vi "Close.vi"(8 "error in (no error)":errorcluster, 11 "LXIPXISwitching in":refnum<class "LXIPXISwitching.lvclass">) -> (0 "error out":errorcluster, 3 "LXIPXISwitching out":refnum<class "LXIPXISwitching.lvclass">)   [LabVIEW 2019, in "LXIPXISwitching.lvclass"]
uses:
  LXIPXISwitching.lvclass
  InstrumentSetup.vi
  InstrControl.lvclass
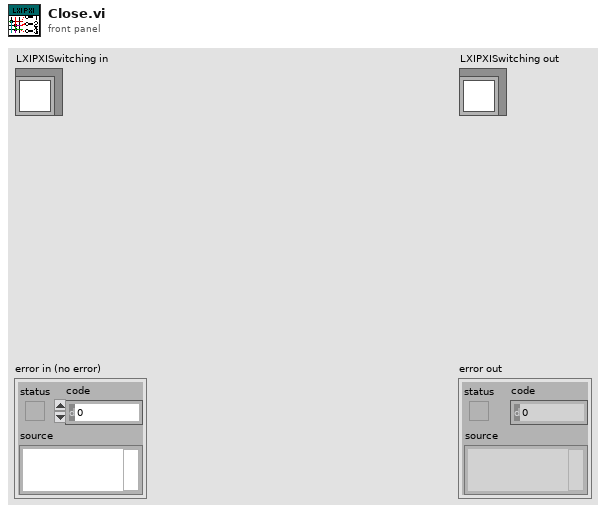
[diagram p1: front panel]
types:
  T1 = cluster{"MUX":string, "Matrix":string, "Breadboard":string, "LXIPXI Switching":refnum<class "LXIPXISwitching.lvclass">, "MUX PN":string, "Matrix  PN":string, "Breadboard PN":string, "MUX ID":string, "Matrix ID":string, "Breadboard ID":string, "LCR?":bool, "SMU?":bool}
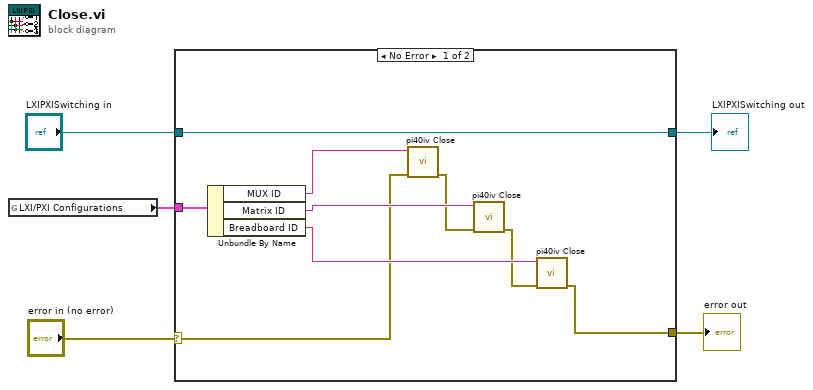
[diagram p0: block diagram]
diagram:
  n1 = global read "InstrumentSetup.vi" "LXI/PXI Configurations"() -> (w4:T1)
  n2 = case shown="No Error" "error in (no error)" {
    selector: "error in (no error)" -> [w10 w16]
    tunnel: w4 -> [w14 _]
    tunnel: [w7 w16] -> w3
    tunnel: [w6 w15] -> w1
    tunnel: "LXIPXISwitching in" -> [w6 w15]
    frame No Error {
      n3 = Unbundle By Name(w14) -> ("MUX ID"=w13:string, "Matrix ID"=w12:string, "Breadboard ID"=w11:string)
      n4 = call <instrlib>:"pi40iv Close.vi"("error in (no error)"=w10, "instrument handle"=w13) -> ("error out"=w9:errorcluster)  [unwired: 9 in]
      n5 = call <instrlib>:"pi40iv Close.vi"("error in (no error)"=w9, "instrument handle"=w12) -> ("error out"=w8:errorcluster)  [unwired: 9 in]
      n6 = call <instrlib>:"pi40iv Close.vi"("error in (no error)"=w8, "instrument handle"=w11) -> ("error out"=w7:errorcluster)  [unwired: 9 in]
    }
    frame Error {
    }
  }
  "error out" <- w3
  "LXIPXISwitching out" <- w1
